vi "LIA Host Filter and Decimation.vi"(0 "I in":dbl[](array[numeric]), 1 "Enable?":bool, 2 "filter in in":T1 {"mSRate_QSettings"."source" items=["Coef a/k"=0, "Coef b/v"=7, "Input"=1, "Output"=2, "Multiplicand"=3, "Product"=4, "Sum"=5, "Delay"=6, "Gain"=8]}, 3 "decimation base in":i32, 7 "Q in":dbl[](array[numeric])) -> (4 "Decimated I":dbl[](array[numeric]), 8 "Decimated Q":dbl[](array[numeric]))   [LabVIEW 2018]
uses:
  <vilib>/addons/Digital Filter Design/_Objects.llb/DFD Filter Obj.ctl
  <vilib>/addons/Digital Filter Design/_Objects.llb/DFD Filter Coef.ctl
  <vilib>/addons/Digital Filter Design/_Objects.llb/DFD Filter Structure Type Selector.ctl
  <vilib>/addons/Digital Filter Design/_Objects.llb/dfd_Internal Quantization Settings.ctl
  <vilib>/addons/Digital Filter Design/_Objects.llb/dfd_Internal Quantization Srcs.ctl
  <vilib>/addons/Digital Filter Design/_Objects.llb/DFD Coef Norm Type.ctl
  <vilib>/addons/Digital Filter Design/Process.llb/DFD Filtering (Array).vi
  <vilib>/Analysis/2dsp.llb/Decimate (continuous, DBL).vi
  <vilib>/addons/Digital Filter Design/NI_DigFilterLicensed.lvlib
  <vilib>/Analysis/NI_AALPro.lvlib
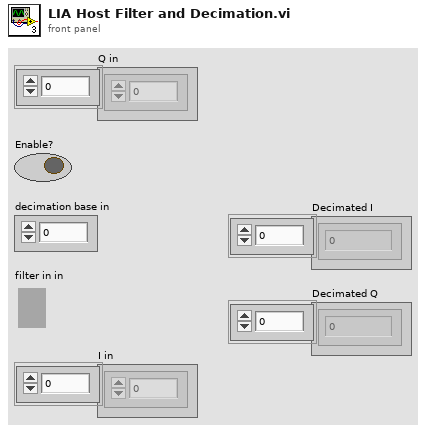
[diagram p1: front panel]
types:
  T1 = typedef "NI_DigFilterLicensed.lvlib/DFD Filter Obj.ctl" = cluster{"mSRate_Fs":dbl, "mSRate_Version":string, "mSRate_Comments":string, "mSRate_OrgCoef":T2, "mSRate_CurCoef":T2, "mSRate_Quantized?":bool, "mSRate_QCoef":T2, "mSRate_QSettings":T4[], "mSRate_Order":i32, "mSRate_Scaling":cluster{"mSRate_ScaleByPowerOf2?":bool, "mSRate_ScaleType":T6}}
  T2 = typedef "NI_DigFilterLicensed.lvlib/DFD Filter Coef.ctl" = cluster{"type":T3, "gain":dbl, "coef a (k)":dbl[], "coef b (v)":dbl[]}
  T3 = typedef "NI_DigFilterLicensed.lvlib/DFD Filter Structure Type Selector.ctl" = enum16{"Undefined", "FIR Direct Form", "FIR Direct Form Transposed", "FIR Symmetric", "FIR Antisymmetric", "IIR Direct Form I", "IIR Direct Form I Transposed", "IIR Direct Form II", "IIR Direct Form II Transposed", "IIR Cascaded Second Order Sections Form I", "IIR Cascaded Second Order Sections Form I Transposed", "IIR Cascaded Second Order Sections Form II", "IIR Cascaded Second Order Sections Form II Transposed", "Lattice Allpass (basic sections)", "Lattice Allpass (one multiplier sections)", "Lattice Allpass (normalized sections)", "Lattice AR (basic sections)", "Lattice AR (one multiplier sections)", "Lattice AR (normalized sections)", "Lattice MA (minimum phase)", "Lattice MA (maximum phase)", "Lattice ARMA (basic sections)", "Lattice ARMA (one multiplier sections)", "Lattice ARMA (normalized sections)"}
  T4 = typedef "NI_DigFilterLicensed.lvlib/dfd_Internal Quantization Settings.ctl" = cluster{"source":T5, "wl":i16, "iwl":i16, "overflow mode":enum16{"Saturation", "Wrap"}, "rounding mode":enum16{"Nearest", "Truncation"}, "signed?":bool}
  T5 = typedef "NI_DigFilterLicensed.lvlib/dfd_Internal Quantization Srcs.ctl" = u16
  T6 = typedef "NI_DigFilterLicensed.lvlib/DFD Coef Norm Type.ctl" = enum16{"No Norm", "Time Domain 1-Norm", "Time Domain 2-Norm", "Time Domain Inf-Norm"}
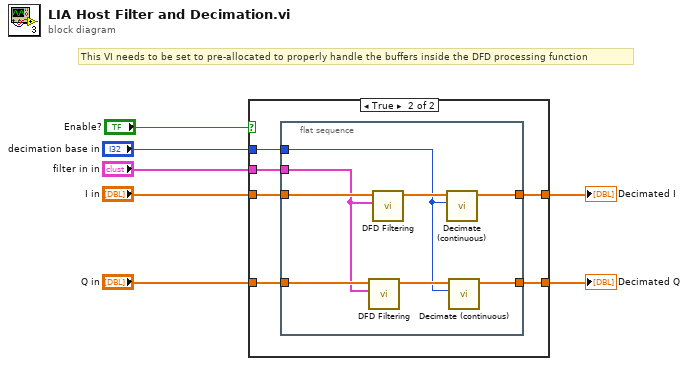
[diagram p0: block diagram]
diagram:
  # "This VI needs to be set to pre-allocated to properly handle the buffers inside the DFD processing function"
  n1 = case shown="True" "Enable?" {
    tunnel: "filter in in" -> [_ w15]
    tunnel: "I in" -> [w9 w14]
    tunnel: "Q in" -> [w8 w13]
    tunnel: [w9 w12] -> w4
    tunnel: [w8 w11] -> w5
    tunnel: "decimation base in" -> [_ w10]
    frame False {
    }
    frame True {
      n2 = flat-sequence {
        tunnel: w15 -> [w17]
        tunnel: [w22] -> w12
        tunnel: [w20] -> w11
        tunnel: w14 -> [w19]
        tunnel: w13 -> [w18]
        tunnel: w10 -> [w16]
        frame #0 {
          n3 = call-poly <vilib>:"DFD Filtering.vi"("filter"=w17, "signal in"=w18) -> ("signal out"=w21:dbl[])  [unwired: 8 in, 1 out]
          n4 = call-poly <vilib>:"DFD Filtering.vi"("filter"=w17, "signal in"=w19) -> ("signal out"=w23:dbl[])  [unwired: 8 in, 1 out]
          n5 = call-poly <vilib>:"Decimate (continuous).vi"("decimating factor"=w16, "X"=w23) -> ("Decimated Array"=w22:dbl[])  [unwired: 8 in, 1 out]
          n6 = call-poly <vilib>:"Decimate (continuous).vi"("decimating factor"=w16, "X"=w21) -> ("Decimated Array"=w20:dbl[])  [unwired: 8 in, 1 out]
        }
      }
    }
  }
  "Decimated Q" <- w5
  "Decimated I" <- w4
